vi "Replace SystemExplorer Project Content.vi"(7 "CDFolderPath String":string, 8 "error in":errorcluster, 9 "System Explorer Project Path":path, 10 "Plugin Name":string, 11 "Template Project path":path) -> (0 "error out":errorcluster)   [LabVIEW 2026, in "NIVS_CDEW_MetaDataObj.lvclass"]
uses:
  NIVS_CDEW_MetaDataObj.lvclass
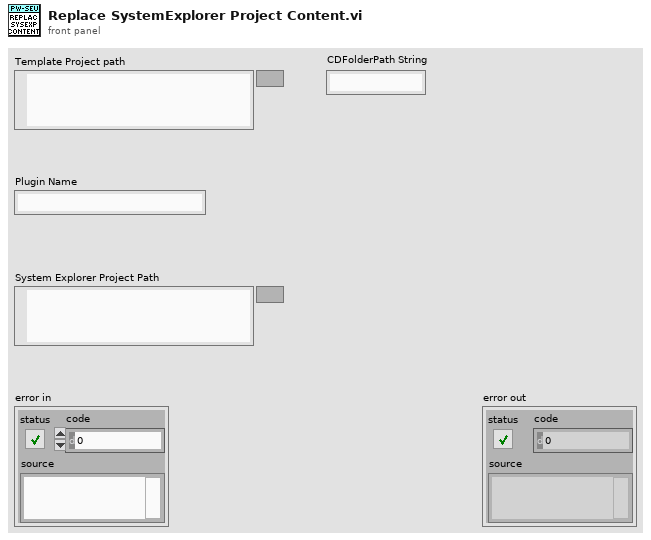
[diagram p1: front panel]
types:
  T1 = enum16{"open", "replace", "create", "open or create", "replace or create", "replace or create with confirmation"}
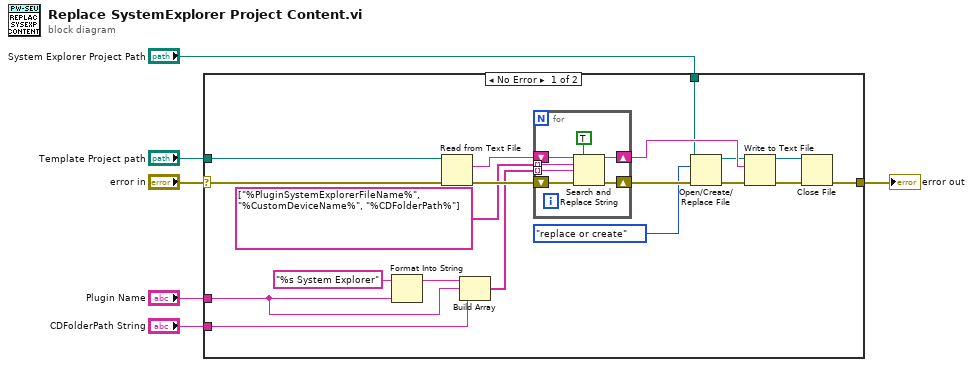
[diagram p0: block diagram]
diagram:
  n1 = case shown="No Error" "error in" {
    selector: "error in" -> [w9 w33]
    tunnel: "Template Project path" -> [w25 _]
    tunnel: [w21 w33] -> w5
    tunnel: "System Explorer Project Path" -> [w16 _]
    tunnel: "Plugin Name" -> [w8 _]
    tunnel: "CDFolderPath String" -> [w7 _]
    frame No Error {
      n2 = Format Into String(format string="%s System Explorer", w8) -> (resulting string=w10:string)  [unwired: 2 in, 1 out]
      n3 = Read from Text File(file (use dialog)=w25, error in=w9) -> (text=w20:string, error out=w23:errorcluster)  [unwired: 2 in, 2 out]
      n4 = Build Array(w10, w8, w7) -> (w18:string[])
      n5 = for {
        shift-right: [w31] -> w24
        shift-left: w23 -> [w30]
        shift-right: [w26] -> w17
        shift-left: w20 -> [w29]
        tunnel: string[] ["%PluginSystemExplorerFileName%", "%CustomDeviceName%", "%CDFolderPath%"] -> [w28] mode=indexing
        tunnel: w18 -> [w27] mode=indexing
        n6 = Search and Replace String(replace all?=TRUE ("replace all? (F)"), input string=w29, search string=w28, replace string=w27, error in=w30) -> (result string=w26:string, error out=w31:errorcluster)  [unwired: 3 in, 2 out]
      }
      n7 = Open/Create/Replace File(file path (use dialog)=w16, error in=w24, operation (0:open)=T1."replace or create") -> (refnum out=w15:refnum<file>, error out=w14:errorcluster)  [unwired: 3 in, 1 out]
      n8 = Write to Text File(file (use dialog)=w15, text=w17, error in=w14) -> (refnum out=w13:refnum<file>, error out=w12:errorcluster)  [unwired: 1 in, 1 out]
      n9 = Close File(refnum=w13, error in=w12) -> (error out=w21:errorcluster)  [unwired: 1 out]
    }
    frame Error {
    }
  }
  "error out" <- w5
